vi "Set RTD Type.vi"(8 "error in (no error)":errorcluster, 10 "RTD Sensor (0: 100 ohm PT385)":u32(ring) items=["100 ohm PT385", "200 ohm PT385", "500 ohm PT385", "1000 ohm PT385", "PT3926", "PT3916", "CU10", "NI120"], 11 "VISA resource name":refnum<visa-resource-name>) -> (0 "error out":errorcluster, 3 "VISA resource name out":refnum<visa-resource-name>)   [LabVIEW 2014, in "Fluke 5XXX Series Multicalibrators.lvlib"]
doc: "This VI sets the Resistance Temperature Detector (RTD) sensor type.\n\nBefore using this VI, select RTD using the FL5XMCAL Set Temp Sensor Type.vi . After using this VI, select the output temperature using the FL5XMCAL Set Output Values.vi. Changes in temperature sensors changes the output to 0 °C. Once set, the Calibrator retains the RTD type until power off or reset.\n\nNote:\n\nThis VI is available only for instrument models 5500A and 5520A."
uses:
  Fluke 5XXX Series Multicalibrators.lvlib
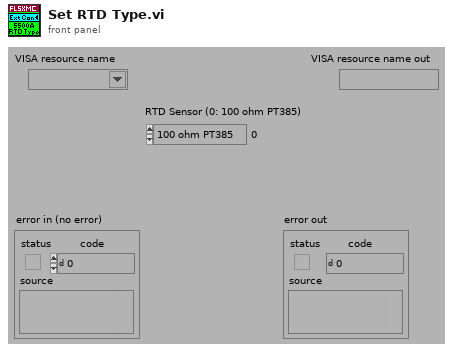
[diagram p1: front panel]
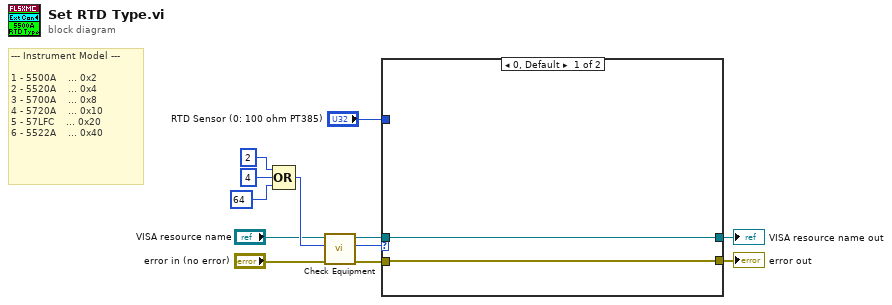
[diagram p0: block diagram]
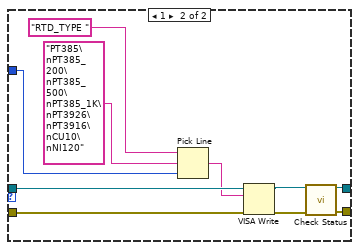
[diagram p2: hidden frame]
diagram:
  # "--- Instrument Model ---\n\n1 - 5500A    ... 0x2\n2 - 5520A    ... 0x4\n3 - 5700A    ... 0x8\n4 - 5720A    ... 0x10\n5 - 57LFC    ... 0x20\n6 - 5522A    ... 0x40"
  n1 = Compound Arithmetic op=OR(2 ("Numeric"), 4 ("Numeric"), 64 ("Numeric")) -> (w9:i32)
  n2 = call "Check Equipment.vi"("error in (no error)"="error in (no error)", "Bit Mask"=w9, "VISA resource name"="VISA resource name") -> ("error out"=w12:errorcluster, "Present?"=w11:u32, "VISA resource name out"=w10:refnum<visa-resource-name>)  [unwired: 6 in]
  n3 = case shown="0, Default" w11 {
    tunnel: "RTD Sensor (0: 100 ohm PT385)" -> [_ w19]
    tunnel: [w13 w15] -> w2
    tunnel: w12 -> [w14 w22]
    tunnel: w10 -> [w13 w21]
    tunnel: [w14 w18] -> w3
    frame 0, Default {
    }
    frame 1 {
      n4 = Pick Line(string ("")="RTD_TYPE " ("Reset Command"), multi-line string="PT385\nPT385_200\nPT385_500\nPT385_1K\nPT3926\nPT3916\nCU10\nNI120", line index=w19) -> (output string=w20:string)
      n5 = VISA Write(VISA resource name=w21, write buffer=w20, error in (no error)=w22) -> (VISA resource name out=w16:refnum<visa-resource-name>, error out=w17:errorcluster)  [unwired: 1 out]
      n6 = call "Check Status.vi"("VISA resource name"=w16, "error in (no error)"=w17) -> ("VISA resource name out"=w15:refnum<visa-resource-name>, "error out"=w18:errorcluster)  [unwired: 12 in]
    }
  }
  "VISA resource name out" <- w2
  "error out" <- w3
